vi "Configure Enable Keypad.vi"(5 "Retry Attempts (0)":i32 min=0, 8 "error in":errorcluster, 11 "VISA resource name":refnum<visa-resource-name>) -> (0 "error out":errorcluster, 3 "VISA resource name out":refnum<visa-resource-name>)   [LabVIEW 2020, in "ChromTech Series III Pump.lvlib"]
doc: "Run the pump."
uses:
  <instrlib>/ChromTech Series III Pump/ChromTech Series III Pump.lvlib
panel:
  out "Response":string
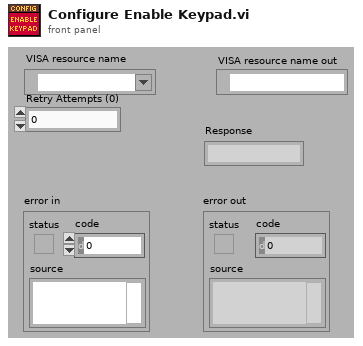
[diagram p1: front panel]
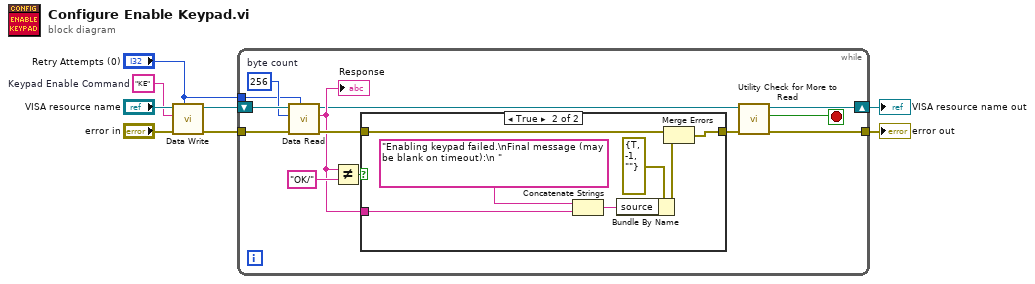
[diagram p0: block diagram]
diagram:
  w5 = "KE"  # Keypad Enable Command
  n1 = call <instrlib>:"Data Write.vi"("Retry Attempts (0)"="Retry Attempts (0)", "error in (no error)"="error in", "Command"=w5, "VISA Refnum in"="VISA resource name") -> ("error out"=w3:errorcluster, "VISA Refnum out"=w7:refnum<visa-resource-name>)  [unwired: 6 in]
  n2 = while {
    tunnel: "Retry Attempts (0)" -> [w13]
    shift-right: [w10] -> w4
    shift-left: w7 -> [w21]
    tunnel: w3 -> [w17]
    tunnel: [w12] -> w2
    stop <- w9 stop-if-true
    w20 = u32 256  # byte count
    n3 = call <instrlib>:"Data Read.vi"("Retry Attempts (0)"=w13, "error in (no error)"=w17, "Bytes to read"=w20, "VISA Refnum in"=w21) -> ("error out"=w15:errorcluster, "read buffer"=w14:string, "VISA Refnum out"=w11:refnum<visa-resource-name>)  [unwired: 5 in]
    "Response" <- w14
    n4 = Not Equal?(x=w14, y="OK/") -> (x != y?=w18:bool)
    n5 = case shown="True" w18 {
      tunnel: [w22 w28] -> w16
      tunnel: w15 -> [w22 w27]
      tunnel: w14 -> [_ w23]
      frame False {
      }
      frame True {
        n6 = Concatenate Strings("Enabling keypad failed.\nFinal message (may be blank on timeout):\n ", w23) -> (w25:string)
        n7 = Bundle By Name(cluster=errorcluster {"status"=TRUE, "code"=-1, "source"=""} ("error out"), "source"=w25) -> (w26:errorcluster)
        n8 = Merge Errors(w27, w26) -> (w28:errorcluster)
      }
    }
    n9 = call <instrlib>:"Utility Check for More to Read.vi"("error in (no error)"=w16, "VISA Refnum in"=w11) -> ("error out (unchanged)"=w12:errorcluster, "More to read?"=w9:bool, "VISA Refnum out"=w10:refnum<visa-resource-name>)  [unwired: 7 in]
  }
  "VISA resource name out" <- w4
  "error out" <- w2
